vi "copyImagesToDataDir.vi"(8 "error in (no error)":errorcluster, 9 "BECRenaming":bool, 10 "ImagePaths in":path[](array[path]), 11 "FileNeologist in":refnum<class "FileNeologist.lvclass">) -> (0 "error out":errorcluster, 2 "ImagePaths out":path[](array[path]), 3 "FileNeologist out":refnum<class "FileNeologist.lvclass">)   [LabVIEW 2011, in "Tools.lvlib" / "Filing.lvlib" / "FileNeologist.lvclass"]
uses:
  FileNeologist.lvclass
  FileNeologist.lvclass/FileNeologist.ctl
panel:
  out "Array":string[](array[string])
  out "scriptName":string
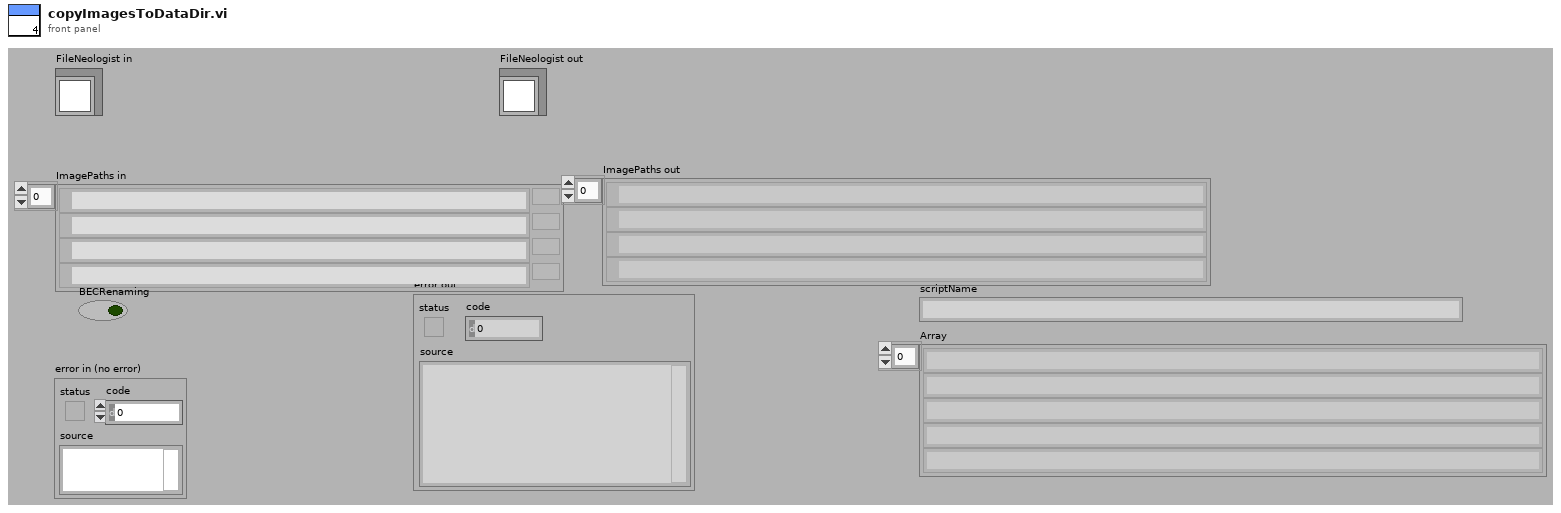
[diagram p1: front panel]
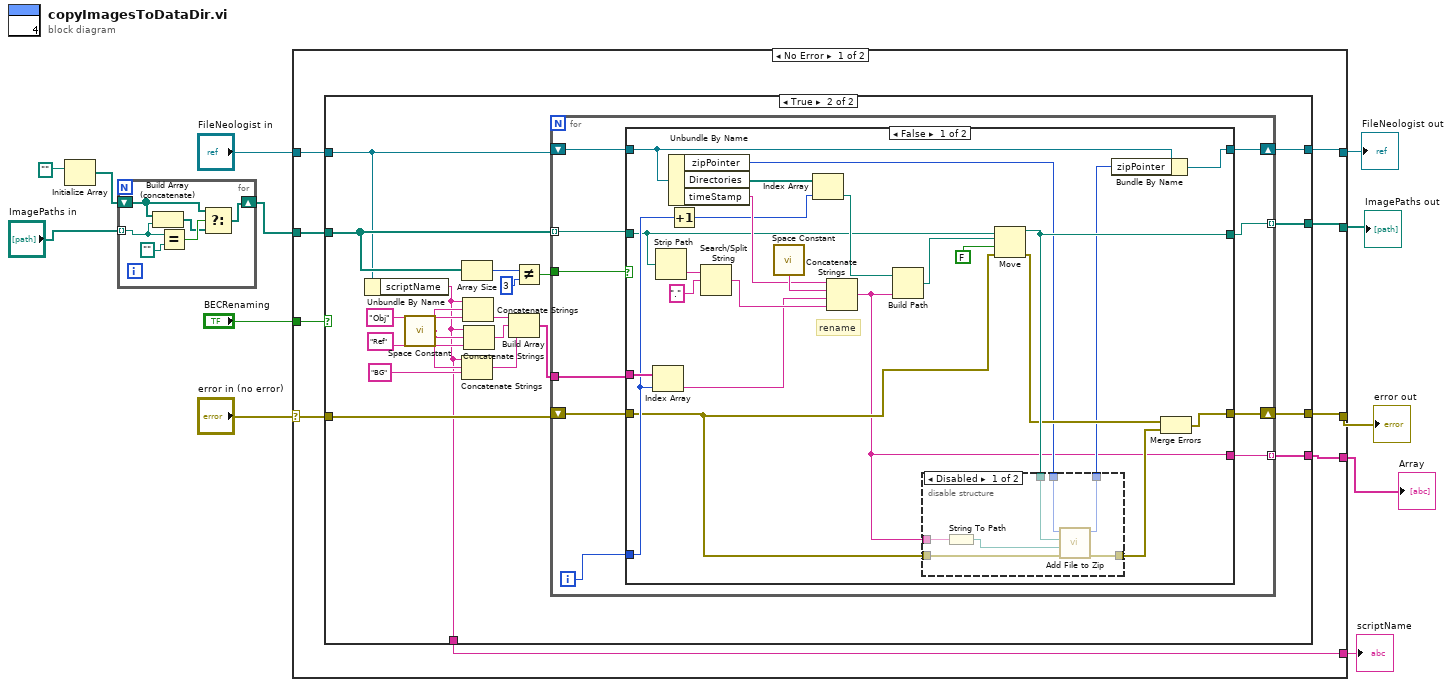
[diagram p0: block diagram]
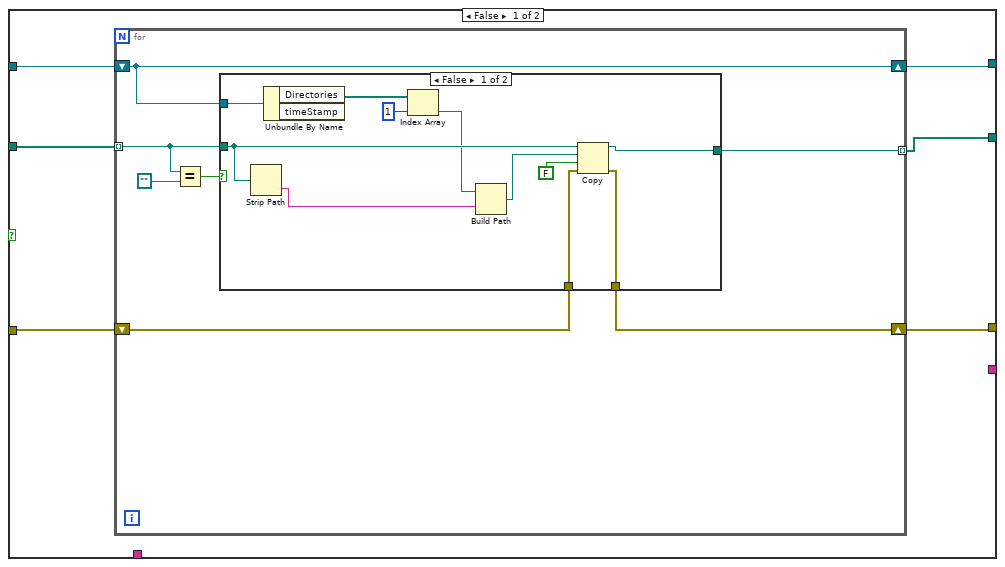
[diagram p2: hidden frame]
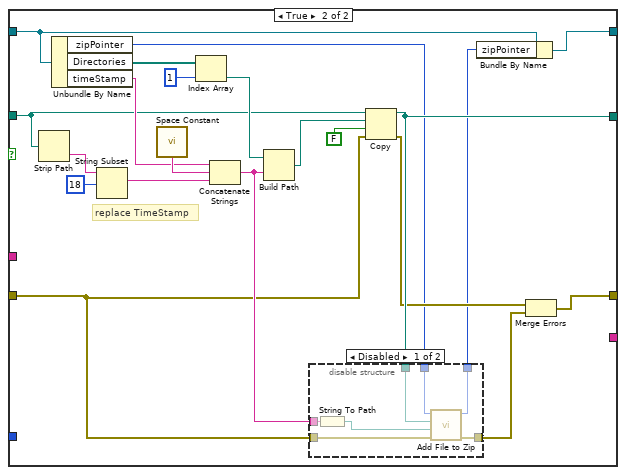
[diagram p5: hidden frame]
diagram:
  n1 = Initialize Array(path "") -> (w5:path[])  [unwired: 1 in]
  n2 = for {
    tunnel: "ImagePaths in" -> [w14] mode=indexing
    shift-right: [w16] -> w3
    shift-left: w5 -> [w15]
    n3 = Build Array (concatenate)(w15, w14) -> (w13:path[])
    n4 = Equal?(x=w14, y=path "") -> (x = y?=w17:bool)
    n5 = Select(t=w15, s=w17, f=w13) -> (s? t:f=w16:path[])
  }
  n6 = case shown="No Error" "error in (no error)" {
    selector: "error in (no error)" -> [w24 w143]
    tunnel: [w26 w143] -> w9
    tunnel: [w25 w142] -> w10
    tunnel: "FileNeologist in" -> [w22 w142]
    tunnel: w3 -> [w23 _]
    tunnel: [w27 _] -> w8
    tunnel: "BECRenaming" -> [w21 _]
    tunnel: [w20 _] -> w2
    tunnel: [w19 _] -> w1
    frame No Error {
      n7 = case shown="True" w21 {
        tunnel: [w30 w72] -> w27
        tunnel: [w29 w71] -> w26
        tunnel: [w28 w70] -> w25
        tunnel: w24 -> [w31 w69]
        tunnel: w23 -> [w32 w67]
        tunnel: w22 -> [w33 w66]
        tunnel: [_ w55] -> w20
        tunnel: [_ w54] -> w19
        frame False {
          n8 = for {
            tunnel: w32 -> [w35] mode=indexing
            shift-right: [w38] -> w28
            shift-left: w33 -> [w38]
            tunnel: [w39] -> w30 mode=indexing
            shift-right: [w37] -> w29
            shift-left: w31 -> [w40]
            n9 = Equal?(x=w35, y=path "") -> (x = y?=w34:bool)
            n10 = case shown="False" w34 {
              tunnel: w35 -> [w51 w53]
              tunnel: w40 -> [w50 w52]
              tunnel: [w49 w53] -> w39
              tunnel: w38 -> [w43 _]
              tunnel: [w42 w52] -> w37
              frame False {
                n11 = Strip Path(path=w51) -> (name=w41:string)  [unwired: 1 out]
                n12 = Unbundle By Name(w43) -> ("Directories"=w46:path[])  [unwired: 1 out]
                n13 = Index Array(array=w46, index=1) -> (element=w45:path)
                n14 = Build Path(base path=w45, name or relative path=w41) -> (appended path=w47:path)
                n15 = Copy(8:w50, 9:FALSE, 10:w47, 11:w51) -> (0:w42:errorcluster, 3:w49:path)  [unwired: 1 in, 1 out]
              }
              frame True {
              }
            }
          }
        }
        frame True {
          n16 = Unbundle By Name(w66) -> ("scriptName"=w55:string)
          n17 = call <vilib>:"Space Constant.vi"() -> ("String"=w59:string)
          n18 = Array Size(array=w67) -> (size(s)=w57:i32)
          n19 = Concatenate Strings(w55, w59, "BG") -> (w62:string)
          n20 = Concatenate Strings(w55, w59, "Obj") -> (w64:string)
          n21 = Concatenate Strings(w55, w59, "Ref") -> (w63:string)
          n22 = Build Array(w64, w63, w62) -> (w68:string[])
          n23 = Not Equal?(x=w57, y=3) -> (x != y?=w56:bool)
          n24 = for {
            tunnel: w67 -> [w82] mode=indexing
            tunnel: [w81] -> w72 mode=indexing
            shift-right: [w78] -> w70
            shift-left: w66 -> [w79]
            shift-right: [w80] -> w71
            shift-left: w69 -> [w77]
            tunnel: w68 -> [w76]
            tunnel: w56 -> [w74]
            tunnel: [w73] -> w54 mode=indexing
            i -> [w75]
            n25 = case shown="False" w74 {
              tunnel: w82 -> [w86 w118]
              tunnel: [w103 w130] -> w81
              tunnel: [w101 w128] -> w80
              tunnel: w79 -> [w95 w122]
              tunnel: [w97 w124] -> w78
              tunnel: w77 -> [w84 w119]
              tunnel: w76 -> [w94 _]
              tunnel: w75 -> [w92 _]
              tunnel: [w83 _] -> w73
              frame False {
                # "rename"
                n26 = Index Array(array=w94, index=w92) -> (element=w87:string)
                n27 = Strip Path(path=w86) -> (name=w90:string)  [unwired: 1 out]
                n28 = Unbundle By Name(w95) -> ("zipPointer"=w96:i32, "Directories"=w102:path[], "timeStamp"=w104:string)
                n29 = Increment(x=w92) -> (x+1=w91:i32)
                n30 = Search/Split String(string=w90, search string/char (-)=".") -> (match + rest of string=w88:string)  [unwired: 1 in, 2 out]
                n31 = call <vilib>:"Space Constant.vi"() -> ("String"=w105:string)
                n32 = Index Array(array=w102, index=w91) -> (element=w93:path)
                n33 = Concatenate Strings(w104, w105, w87, w88) -> (w83:string)
                n34 = Build Path(base path=w93, name or relative path=w83) -> (appended path=w85:path)
                n35 = Move(source path=w86, error in=w84, 9:FALSE, 10:w85) -> (error out=w100:errorcluster, 3:w103:path)  [unwired: 1 in, 1 out]
                n36 = disable-structure shown="Disabled" {
                  disable-tunnel: w103 -> [w113 _]
                  disable-tunnel: [w111 _] -> w99
                  disable-tunnel: [w110 _] -> w98
                  disable-tunnel: w96 -> [w109 _]
                  disable-tunnel: w83 -> [w108 _]
                  disable-tunnel: w84 -> [w107 _]
                  frame Disabled {
                    n37 = String To Path(string=w108) -> (path=w112:path)
                    n38 = call <vilib>:"Add File to Zip.vi"("error in (no error)"=w107, "destination path in zip"=w112, "source file path"=w113, "zip file in"=w109) -> ("error out"=w111:errorcluster, "zip file out"=w110:i64)  [unwired: 6 in]
                  }
                  frame Enabled {
                  }
                }
                n39 = Bundle By Name(cluster=w95, "zipPointer"=w98) -> (w97:refnum<class "FileNeologist.lvclass">)
                n40 = Merge Errors(w100, w99) -> (w101:errorcluster)
              }
              frame True {
                # "replace TimeStamp"
                n41 = Strip Path(path=w118) -> (name=w116:string)  [unwired: 1 out]
                n42 = Unbundle By Name(w122) -> ("zipPointer"=w123:i32, "Directories"=w129:path[], "timeStamp"=w131:string)
                n43 = String Subset(string=w116, offset (0)=18) -> (substring=w115:string)  [unwired: 1 in]
                n44 = call <vilib>:"Space Constant.vi"() -> ("String"=w133:string)
                n45 = Index Array(array=w129, index=1) -> (element=w120:path)
                n46 = Concatenate Strings(w131, w133, w115) -> (w121:string)
                n47 = Build Path(base path=w120, name or relative path=w121) -> (appended path=w132:path)
                n48 = Copy(8:w119, 9:FALSE, 10:w132, 11:w118) -> (0:w127:errorcluster, 3:w130:path)  [unwired: 1 in, 1 out]
                n49 = disable-structure shown="Disabled" {
                  disable-tunnel: w130 -> [w141 _]
                  disable-tunnel: [w139 _] -> w126
                  disable-tunnel: [w138 _] -> w125
                  disable-tunnel: w123 -> [w137 _]
                  disable-tunnel: w121 -> [w136 _]
                  disable-tunnel: w119 -> [w135 _]
                  frame Disabled {
                    n50 = String To Path(string=w136) -> (path=w140:path)
                    n51 = call <vilib>:"Add File to Zip.vi"("error in (no error)"=w135, "destination path in zip"=w140, "source file path"=w141, "zip file in"=w137) -> ("error out"=w139:errorcluster, "zip file out"=w138:i64)  [unwired: 6 in]
                  }
                  frame Enabled {
                  }
                }
                n52 = Bundle By Name(cluster=w122, "zipPointer"=w125) -> (w124:refnum<class "FileNeologist.lvclass">)
                n53 = Merge Errors(w127, w126) -> (w128:errorcluster)
              }
            }
          }
        }
      }
    }
    frame Error {
    }
  }
  "error out" <- w9
  "FileNeologist out" <- w10
  "ImagePaths out" <- w8
  "scriptName" <- w2
  "Array" <- w1
